vi "_compute_32bit_AckID.vi"(11 "ControlPacket in":refnum<class "ControlPacket.lvclass">) -> (3 "ACK ID":u32)   [LabVIEW 2013, in "MQTT Base.lvlib" / "Session.lvclass"]
uses:
  Session.lvclass
  <vilib>/LabVIEW Open Source Project/MQTT Control Packets/Control Packets/ControlPacket/ControlPacket.lvclass
  <vilib>/LabVIEW Open Source Project/MQTT Control Packets/Control Packets/ControlPacket/ControlPacket.lvclass/ControlPacket.ctl
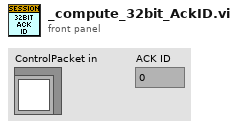
[diagram p1: front panel]
types:
  T1 = typedef "MQTT_Control_Packets.lvlib/ControlPacket.lvclass/Control Packet Type -- enum.ctl" = enum16{"Reserved", "CONNECT", "CONNACK", "PUBLISH", "PUBACK", "PUBREC", "PUBREL", "PUBCOMP", "SUBSCRIBE", "SUBACK", "UNSUBSCRIBE", "UNSUBACK", "PINGREQ", "PINGRESP", "DISCONNECT", "AUTH"}
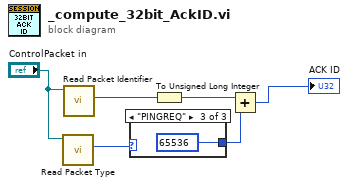
[diagram p0: block diagram]
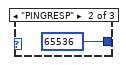
[diagram p3: hidden frame]
diagram:
  n1 = call <vilib>:"Read Packet Type.vi"("ControlPacket in"="ControlPacket in") -> ("Control Packet Type"=w5:T1)  [unwired: 9 in, 1 out]
  n2 = call <vilib>:"Read Packet Identifier.vi"("ControlPacket in"="ControlPacket in") -> ("Packet Identifier"=w4:u16)  [unwired: 8 in, 2 out]
  n3 = case shown="\"PINGREQ\"" w5 {
    tunnel: [_ u32 65536 u32 65536] -> w2
    frame Default {
    }
    frame "PINGRESP" {
    }
    frame "PINGREQ" {
    }
  }
  n4 = To Unsigned Long Integer(number=w4) -> (unsigned 32bit integer=w3:u32)
  n5 = Add(x=w3, y=w2) -> (x+y=→"ACK ID":u32)
